vi "to INT64.vi"(8 "error in":errorcluster, 11 "byte":u8[](array[numeric]) format="%b") -> (0 "error out":errorcluster, 2 "INT64":i64, 3 "remaining bytes":u8[](array[numeric]))   [LabVIEW 2020, in "MessagePack.lvlib" / "MessagePack.lvclass"]
uses:
  MessagePack.lvclass
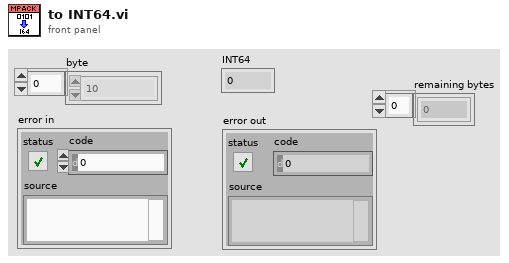
[diagram p1: front panel]
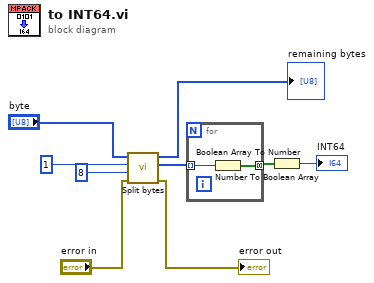
[diagram p0: block diagram]
diagram:
  n1 = call "Split bytes.vi"("error in"="error in", "End index"=8 ("length"), "Start index"=1 ("index"), "bytes in"="byte") -> ("error out"=→"error out":errorcluster, "selected bytes"=w4:u8[], "remaining bytes"=→"remaining bytes":u8[])  [unwired: 4 in, 1 out]
  n2 = for {
    tunnel: w4 -> [w11] mode=indexing
    tunnel: [w10] -> w8 mode=concatenating
    n3 = Number To Boolean Array(number=w11) -> (Boolean array=w10:bool[])
  }
  n4 = Boolean Array To Number(Boolean array=w8) -> (number=→"INT64":i64)
